vi "Adv_Support_SPEtoDataArray.vi"(8 "error in (no error)":errorcluster, 9 "ROI Info":T3={"ROI Height"=[0], "ROI Width"=[], "ROI Stride"=[], "ROI Size"=[]}, 10 "Frame Info":T2, 11 "SPE Refnum":refnum<file>) -> (0 "error out":errorcluster, 2 "Data":T1(array[cluster]), 3 "SPE Refnum 2":refnum<file>)   [LabVIEW 2020, in "LightField Automation.lvclass"]
uses:
  LightField Automation.lvclass
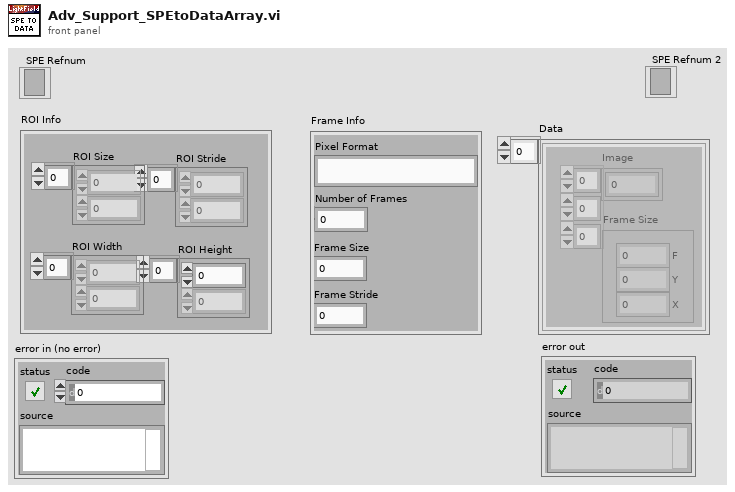
[diagram p1: front panel]
types:
  T1 = cluster{"Image":dbl[][][], "Frame Size":cluster{"F":i32, "Y":i32, "X":i32}}[]
  T2 = cluster{"Pixel Format":string, "Number of Frames":i32, "Frame Size":i32, "Frame Stride":i64}
  T3 = cluster{"ROI Height":i32[], "ROI Width":i32[], "ROI Stride":i32[], "ROI Size":i64[]}
  T4 = cluster{"Image":dbl[][][], "Frame Size":cluster{"F":i32, "Y":i32, "X":i32}}
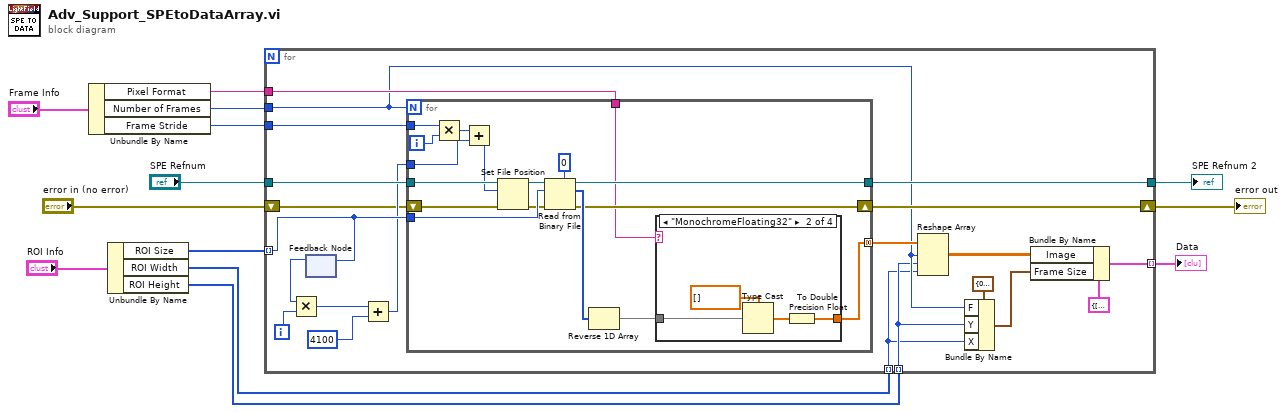
[diagram p0: block diagram]
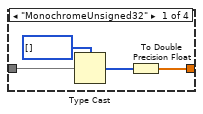
[diagram p2: hidden frame]
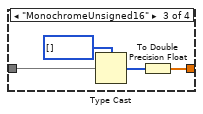
[diagram p3: hidden frame]
diagram:
  n1 = Unbundle By Name("Frame Info") -> ("Pixel Format"=w12:string, "Number of Frames"=w1:i32, "Frame Stride"=w2:i64)
  n2 = Unbundle By Name("ROI Info") -> ("ROI Size"=w8:i64[], "ROI Width"=w4:i32[], "ROI Height"=w3:i32[])
  n3 = for {
    tunnel: w8 -> [w29] mode=indexing
    tunnel: "SPE Refnum" -> [w31]
    tunnel: w1 -> [w20]
    tunnel: w2 -> [w33]
    tunnel: w4 -> [w18] mode=indexing
    tunnel: w3 -> [w19] mode=indexing
    tunnel: [w27] -> w9
    shift-right: [w23] -> w11
    shift-left: "error in (no error)" -> [w24]
    tunnel: w12 -> [w22]
    tunnel: [w14] -> w13 mode=indexing
    i -> [w34]
    n4 = feedback-in #1(w29) -> ()
    n5 = feedback #1() -> (w28:i64)  [unwired: 1 in]
    n6 = Multiply(x=w28, y=w34) -> (x*y=w30:i64)
    n7 = Add(x=w30, y=i64 4100) -> (x+y=w25:i64)
    n8 = for {
      N: w20 -> [_]
      tunnel: w31 -> [w51]
      tunnel: w29 -> [w48]
      tunnel: w33 -> [w43]
      tunnel: [w35] -> w32 mode=concatenating
      tunnel: [w44] -> w27
      tunnel: w25 -> [w41]
      shift-right: [w38] -> w23
      shift-left: w24 -> [w39]
      tunnel: w22 -> [w36]
      i -> [w42]
      n9 = Multiply(x=w43, y=w42) -> (x*y=w46:i64)
      n10 = Add(x=w46, y=w41) -> (x+y=w45:i64)
      n11 = Set File Position(offset (in bytes) (0)=w45, refnum=w51, error in=w39) -> (refnum out=w49:refnum<file>, error out=w40:errorcluster)  [unwired: 1 in]
      n12 = Read from Binary File(5:u8 0, 8:w40, 10:w48, 11:w49) -> (0:w38:errorcluster, 2:w47:u8[], 3:w44:refnum<file>)  [unwired: 2 in, 1 out]
      n13 = Reverse 1D Array(array=w47) -> (reversed array=w37:u8[])
      n14 = case shown="\"MonochromeFloating32\"" w36 {
        tunnel: w37 -> [w54 w58 w62 _]
        tunnel: [w52 w56 w60 _] -> w35
        frame "MonochromeUnsigned32" {
          n15 = Type Cast(type=u32[] [], x=w54) -> (*(type *) &x=w53:u32[])
          n16 = To Double Precision Float(number=w53) -> (double precision float=w52:dbl[])
        }
        frame "MonochromeFloating32" {
          n17 = Type Cast(type=sgl[] [], x=w58) -> (*(type *) &x=w57:sgl[])
          n18 = To Double Precision Float(number=w57) -> (double precision float=w56:dbl[])
        }
        frame "MonochromeUnsigned16" {
          n19 = Type Cast(type=u16[] [], x=w62) -> (*(type *) &x=w61:u16[])
          n20 = To Double Precision Float(number=w61) -> (double precision float=w60:dbl[])
        }
        frame Default {
        }
      }
    }
    n21 = Reshape Array(w32, w20, w19, w18) -> (w16:dbl[][][])
    n22 = Bundle By Name(cluster=cluster{"F":i32, "Y":i32, "X":i32} {"F"=0, "Y"=0, "X"=0} ("Frame Size"), "F"=w20, "Y"=w19, "X"=w18) -> (w15:cluster{"F":i32, "Y":i32, "X":i32})
    n23 = Bundle By Name(cluster=T4 {"Image"=[], "Frame Size"={"F"=0, "Y"=0, "X"=0}} ("Cluster"), "Image"=w16, "Frame Size"=w15) -> (w14:T4)
  }
  "Data" <- w13
  "SPE Refnum 2" <- w9
  "error out" <- w11
